vi "AB_1200_1100_Project_Build_Info.vi"(7 "action":T1, 8 "error in (no error)":errorcluster, 10 "buildInfo in":T2, 11 "Object In":T3) -> (0 "error out":errorcluster, 2 "buildInfo out":T2, 3 "Object Out":T3)   [LabVIEW 2020]
uses:
  <vilib>/AppBuilder/RW_Project/AB_RW_Project_PropBag_Action.ctl
  <resource>/Framework/Providers/API/ItemRef.ctl
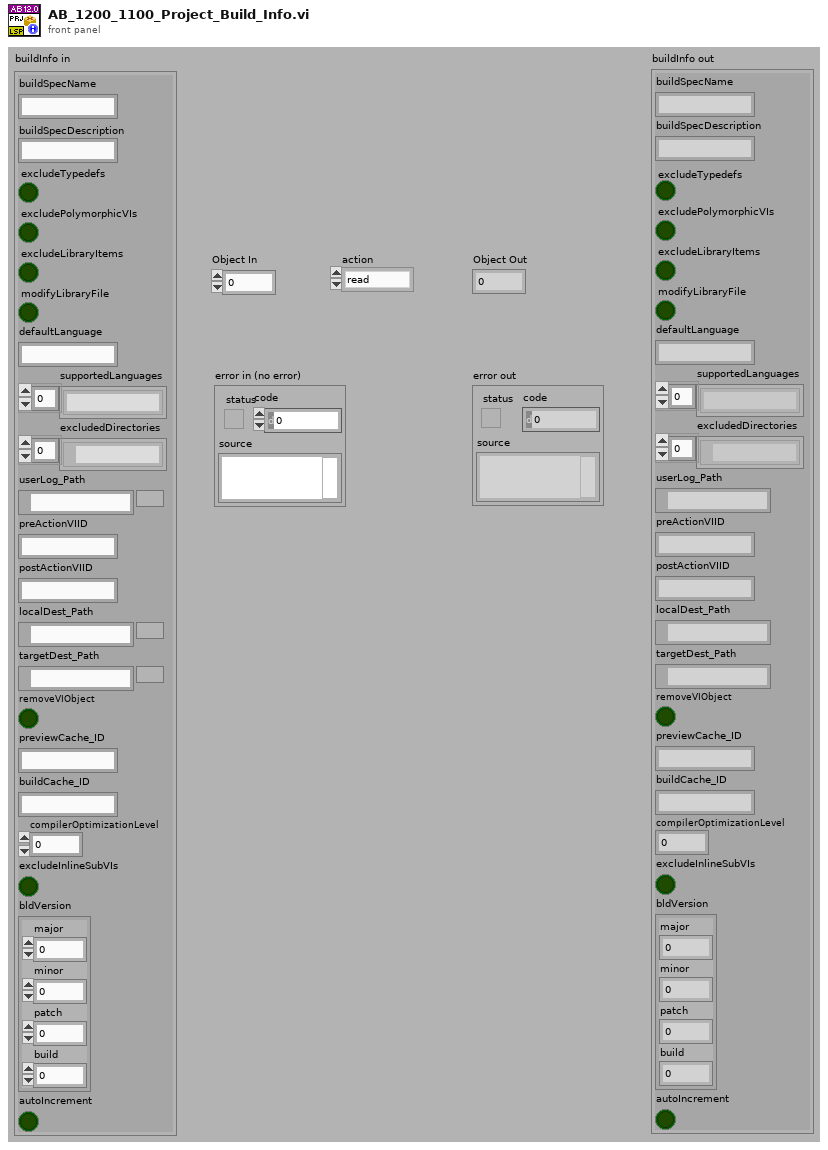
[diagram p1: front panel]
types:
  T1 = typedef "AB_RW_Project_PropBag_Action.ctl" = enum16{"read", "write", "clear", "readPrevious", "writePrevious", "clearPrevious"}
  T2 = cluster{"buildSpecName":string, "buildSpecDescription":string, "excludeTypedefs":bool, "excludePolymorphicVIs":bool, "excludeLibraryItems":bool, "modifyLibraryFile":bool, "defaultLanguage":string, "supportedLanguages":string[], "excludedDirectories":path[], "userLog_Path":path, "preActionVIID":string, "postActionVIID":string, "localDest_Path":path, "targetDest_Path":path, "removeVIObject":bool, "previewCache_ID":string, "buildCache_ID":string, "compilerOptimizationLevel":u32, "excludeInlineSubVIs":bool, "bldVersion":cluster{"major":u16, "minor":u16, "patch":u16, "build":u16}, "autoIncrement":bool}
  T3 = typedef "ItemRef.ctl" = u64
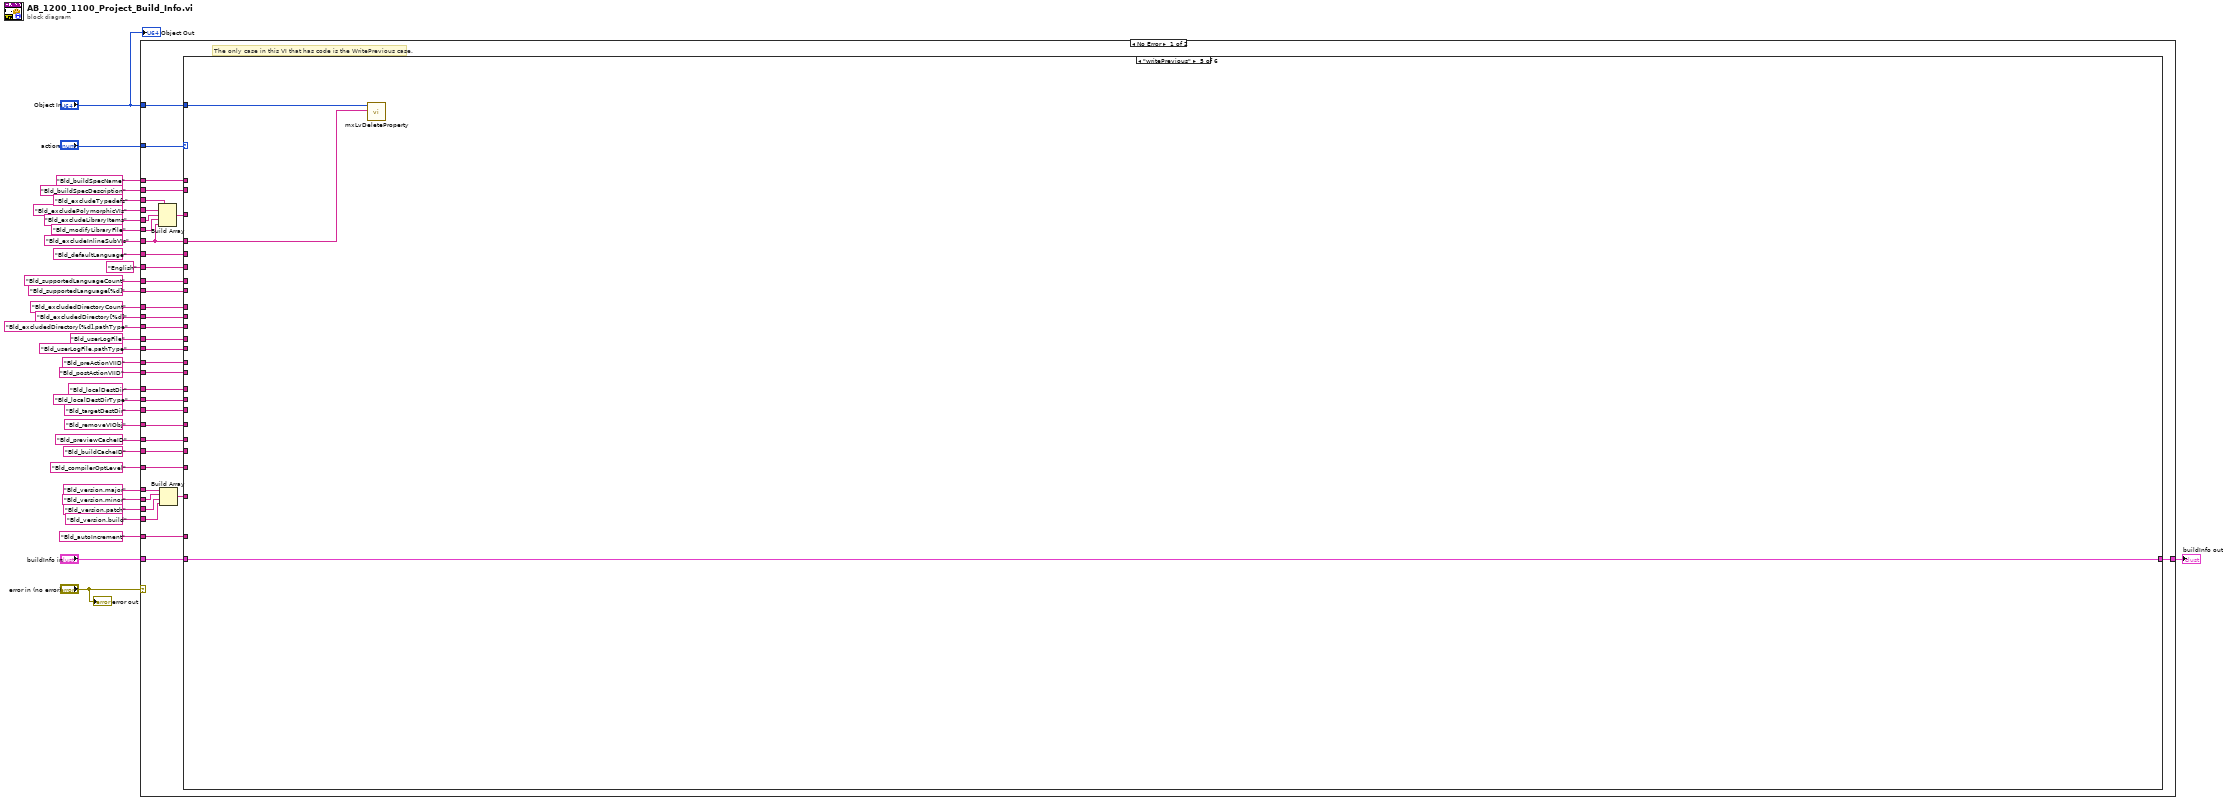
[diagram p0: block diagram]
diagram:
  n1 = case shown="No Error" "error in (no error)" {
    tunnel: "Object In" -> [w71 _]
    tunnel: [w60 _] -> w33
    tunnel: "Bld_buildSpecDescription" ("Tag") -> [w70 _]
    tunnel: "Bld_excludeTypedefs" ("Tag") -> [w56 _]
    tunnel: "Bld_defaultLanguage" ("Tag") -> [w69 _]
    tunnel: "English" ("Tag") -> [w68 _]
    tunnel: "Bld_supportedLanguageCount" ("Tag") -> [w67 _]
    tunnel: "Bld_supportedLanguage[%d]" ("Tag") -> [w66 _]
    tunnel: "Bld_excludedDirectoryCount" ("Tag") -> [w65 _]
    tunnel: "Bld_excludedDirectory[%d]" ("Tag") -> [w64 _]
    tunnel: "Bld_excludedDirectory[%d].pathType" ("Tag") -> [w63 _]
    tunnel: "buildInfo in" -> [w62 _]
    tunnel: "action" -> [w61 _]
    tunnel: "Bld_excludePolymorphicVIs" ("Tag") -> [w59 _]
    tunnel: "Bld_excludeLibraryItems" ("Tag") -> [w58 _]
    tunnel: "Bld_modifyLibraryFile" ("Tag") -> [w57 _]
    tunnel: "Bld_buildSpecName" ("Tag") -> [w54 _]
    tunnel: "Bld_userLogFile" ("Tag") -> [w53 _]
    tunnel: "Bld_userLogFile.pathType" ("Tag") -> [w52 _]
    tunnel: "Bld_preActionVIID" ("Tag") -> [w51 _]
    tunnel: "Bld_postActionVIID" ("Tag") -> [w50 _]
    tunnel: "Bld_localDestDir" ("Tag") -> [w49 _]
    tunnel: "Bld_targetDestDir" ("Tag") -> [w48 _]
    tunnel: "Bld_localDestDirType" ("Tag") -> [w47 _]
    tunnel: "Bld_removeVIObj" ("Tag") -> [w46 _]
    tunnel: "Bld_previewCacheID" ("Tag") -> [w45 _]
    tunnel: "Bld_buildCacheID" ("Tag") -> [w44 _]
    tunnel: "Bld_compilerOptLevel" ("Tag") -> [w43 _]
    tunnel: "Bld_excludeInlineSubVIs" ("Tag") -> [w42 _]
    tunnel: "Bld_version.major" ("Tag") -> [w40 _]
    tunnel: "Bld_version.minor" ("Tag") -> [w39 _]
    tunnel: "Bld_version.patch" ("Tag") -> [w37 _]
    tunnel: "Bld_version.build" ("Tag") -> [w38 _]
    tunnel: "Bld_autoIncrement" ("Tag") -> [w41 _]
    frame No Error {
      # "The only case in this VI that has code is the WritePrevious case."
      n2 = Build Array(w56, w59, w58, w57, w42) -> (w55:string[])
      n3 = Build Array(w40, w39, w37, w38) -> (w36:string[])
      n4 = case shown="\"writePrevious\"" w61 {
        tunnel: w71 -> [_ _ _ _ w77 _]
        tunnel: w70 -> [_ _ _ _ _ _]
        tunnel: w69 -> [_ _ _ _ _ _]
        tunnel: w68 -> [_ _ _ _ _ _]
        tunnel: w67 -> [_ _ _ _ _ _]
        tunnel: w66 -> [_ _ _ _ _ _]
        tunnel: w65 -> [_ _ _ _ _ _]
        tunnel: w64 -> [_ _ _ _ _ _]
        tunnel: w63 -> [_ _ _ _ _ _]
        tunnel: w62 -> [w72 w73 w74 w75 w78 w79]
        tunnel: [w72 w73 w74 w75 w78 w79] -> w60
        tunnel: w55 -> [_ _ _ _ _ _]
        tunnel: w54 -> [_ _ _ _ _ _]
        tunnel: w53 -> [_ _ _ _ _ _]
        tunnel: w52 -> [_ _ _ _ _ _]
        tunnel: w51 -> [_ _ _ _ _ _]
        tunnel: w50 -> [_ _ _ _ _ _]
        tunnel: w49 -> [_ _ _ _ _ _]
        tunnel: w48 -> [_ _ _ _ _ _]
        tunnel: w47 -> [_ _ _ _ _ _]
        tunnel: w46 -> [_ _ _ _ _ _]
        tunnel: w45 -> [_ _ _ _ _ _]
        tunnel: w44 -> [_ _ _ _ _ _]
        tunnel: w43 -> [_ _ _ _ _ _]
        tunnel: w42 -> [_ _ _ _ w76 _]
        tunnel: w41 -> [_ _ _ _ _ _]
        tunnel: w36 -> [_ _ _ _ _ _]
        frame "read" {
        }
        frame "write" {
        }
        frame "clear" {
        }
        frame "readPrevious" {
        }
        frame "writePrevious" {
          n5 = call <resource>:"mxLvDeleteProperty.vi"("Tag"=w76, "Item"=w77) -> ()  [unwired: 1 in, 9 out]
        }
        frame "clearPrevious" {
        }
      }
    }
    frame Error {
    }
  }
  "buildInfo out" <- w33
  "Object Out" <- "Object In"
  "error out" <- "error in (no error)"
